vi "Programacion 9 Lester Roche.vi"() -> ()   [LabVIEW 2011]
panel:
  in  "On/off prg":bool
  out "TemMin":dbl
  out "TempMaxima":dbl
  out "Temperatura promedio":dbl
  in  "On/off A/C":bool
  out "A/C on":bool
  in  "Temperatura deseada":dbl
  out "Temeperatura":i32(slide) scale=0.0..50.0
  # "El programa simula el funcionamiento de un a/c \ndonde se ingresa la temperatura deseada y cada\nvez que la temperatura deseada sea mayor a \ntemperatura no se enciende el compresor del\na/c, pero cuando esta sea menor se enciende el compresor\npero esto solo puede ocurrir siempre el a/c este\nencendido, el programa termina solo cuando decidimos \nnosotros terminar."
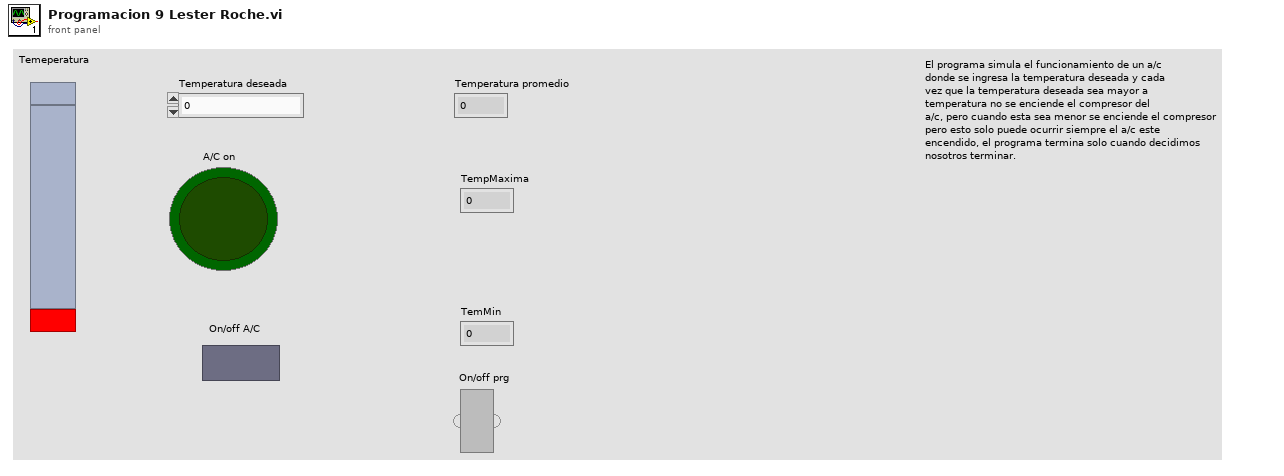
[diagram p1: front panel]
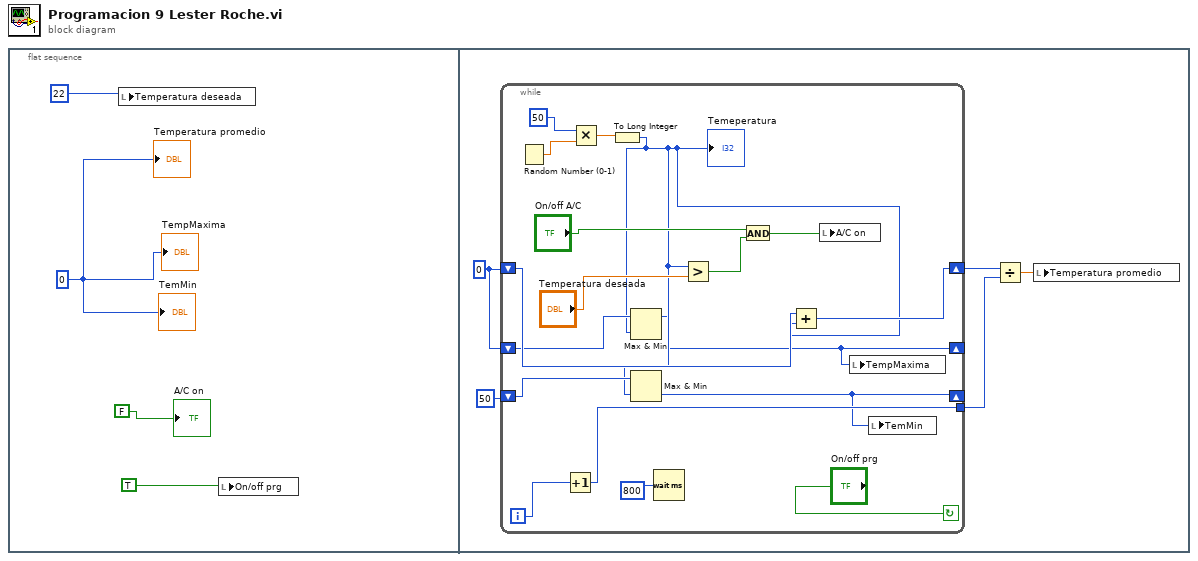
[diagram p0: block diagram]
diagram:
  n1 = flat-sequence {
    frame #0 {
      w4 = 0
      n2 = local write "Temperatura deseada"(22) -> ()
      n3 = local write "On/off prg"(TRUE) -> ()
      "A/C on" <- FALSE
      "TemMin" <- w4
      "TempMaxima" <- w4
      "Temperatura promedio" <- w4
    }
    frame #1 {
      w6 = 0
      n4 = while {
        tunnel: [w17] -> w8
        shift-right: [w15] -> w7
        shift-left: w6 -> [w16]
        shift-right: [w11] -> _
        shift-left: w6 -> [w14]
        shift-right: [w10] -> _
        shift-left: 50 -> [w13]
        i -> [w18]
        stop <- "On/off prg" continue-if-true
        n5 = Random Number (0-1)() -> (number: 0 to 1=w25:dbl)
        n6 = Increment(x=w18) -> (x+1=w17:i32)
        n7 = Multiply(x=50, y=w25) -> (x*y=w24:dbl)
        n8 = To Long Integer(number=w24) -> (32bit integer=w12:i32)
        "Temeperatura" <- w12
        n9 = Max & Min(x=w14, y=w12) -> (max(x,y)=w11:i32)  [unwired: 1 out]
        n10 = Max & Min(x=w13, y=w12) -> (min(x,y)=w10:i32)  [unwired: 1 out]
        n11 = Wait (ms)(milliseconds to wait=800) -> ()  [unwired: 1 out]
        n12 = Greater?(x=w12, y="Temperatura deseada") -> (0:w20:bool)
        n13 = And(x="On/off A/C", y=w20) -> (x .and. y?=w19:bool)
        n14 = Add(x=w16, y=w12) -> (x+y=w15:i32)
        n15 = local write "A/C on"(w19) -> ()
        n16 = local write "TempMaxima"(w11) -> ()
        n17 = local write "TemMin"(w10) -> ()
      }
      n18 = Divide(x=w7, y=w8) -> (x/y=w9:dbl)
      n19 = local write "Temperatura promedio"(w9) -> ()
    }
  }
